vi "S7COMM - Timestamp to DTL.vi"(11 "Time Stamp":timestamp) -> (1 "DTL":T1 {"Weekday" items=["Sunday"=1, "Monday"=2, "Tuesday"=3, "Wednesday"=4, "Thursday"=5, "Friday"=6, "Saturday"=7]; "Month" items=["Jan"=1, "Feb"=2, "Mar"=3, "Apr"=4, "May"=5, "Jun"=6, "Jul"=7, "Aug"=8, "Sep"=9, "Oct"=10, "Nov"=11, "Dec"=12]}, 3 "S7 DTL":u32[](array[numeric]))   [LabVIEW 2014, in "S7NetCom.lvclass"]
uses:
  S7NetCom.lvclass
  S7COMM - DTL--cluster.ctl
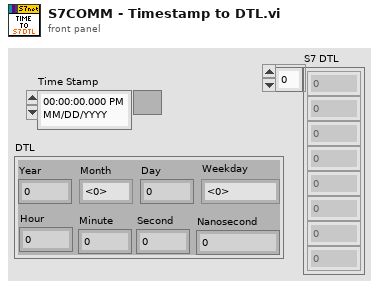
[diagram p1: front panel]
types:
  T1 = typedef "S7NetCom.lvclass/S7COMM - DTL--cluster.ctl" = cluster{"Year":u16, "Month":u8, "Day":u8, "Hour":u8, "Minute":u8, "Second":u8, "Nanosecond":u32, "Weekday":u8}
  T2 = typedef "LVDateTimeRec.ctl" = cluster{"fractional second":dbl, "second":i32, "minute":i32, "hour":i32, "day of month":i32, "month":i32, "year":i32, "day of week":i32, "day of year":i32, "DST":i32}
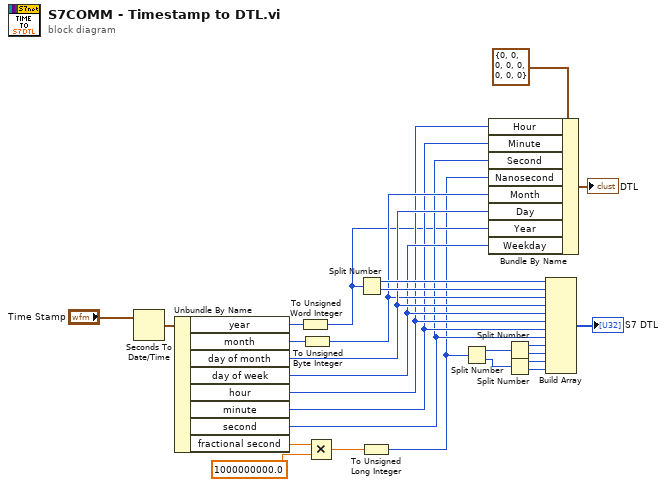
[diagram p0: block diagram]
diagram:
  n1 = Seconds To Date/Time(time stamp (now)="Time Stamp") -> (date time rec=w14:T2)  [unwired: 1 in]
  n2 = Unbundle By Name(w14) -> ("year"=w13:i32, "month"=w12:i32, "day of month"=w11:i32, "day of week"=w9:i32, "hour"=w8:i32, "minute"=w7:i32, "second"=w6:i32, "fractional second"=w5:dbl)
  n3 = To Unsigned Word Integer(number=w13) -> (unsigned 16bit integer=w2:u16)
  n4 = To Unsigned Byte Integer(number=w12) -> (unsigned 8bit integer=w10:u8)
  n5 = Multiply(x=w5, y=1000000000.0) -> (x*y=w3:dbl)
  n6 = Split Number(x=w2) -> (hi(x)=w24:u8, lo(x)=w23:u8)
  n7 = To Unsigned Long Integer(number=w3) -> (unsigned 32bit integer=w1:u32)
  n8 = Split Number(x=w1) -> (hi(x)=w20:u16, lo(x)=w21:u16)
  n9 = Bundle By Name(cluster=T1 {"Year"=0, "Month"=0, "Day"=0, "Hour"=0, "Minute"=0, "Second"=0, "Nanosecond"=0, "Weekday"=0} ("S7 Date & Time"), "Hour"=w8, "Minute"=w7, "Second"=w6, "Nanosecond"=w1, "Month"=w10, "Day"=w11, "Year"=w2, "Weekday"=w9) -> (→"DTL":T1)
  n10 = Split Number(x=w20) -> (hi(x)=w19:u8, lo(x)=w18:u8)
  n11 = Split Number(x=w21) -> (hi(x)=w17:u8, lo(x)=w16:u8)
  n12 = Build Array(w24, w23, w10, w11, w9, w8, w7, w6, w19, w18, w17, w16) -> (→"S7 DTL":i32[])
